vi "myRIO_BRig_RT_TCP__buildStr_initBlock.vi"(7 "input_countTrial":u16, 9 "input_spout":enum16{"Left", "Right"}(ring), 10 "input_iTrial":u16, 11 "input_iBlock":u16) -> (3 "output_str_initBlock":string)   [LabVIEW 2014]
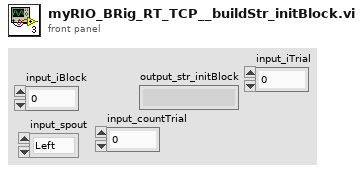
[diagram p1: front panel]
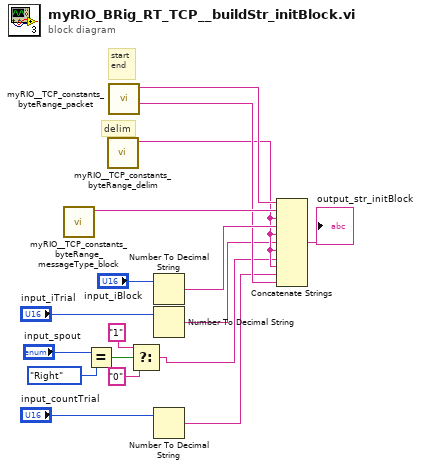
[diagram p0: block diagram]
diagram:
  # "start\nend"
  # "delim"
  n1 = call "myRIO__TCP_constants_byteRange_messageType_block.vi"() -> ("output_Block_char"=w13:string)  [unwired: 10 in, 1 out]
  n2 = Equal?(x="input_spout", y=enum16{"Left", "Right"}."Right") -> (x = y?=w4:bool)
  n3 = call "myRIO__TCP_constants_byteRange_delim.vi"() -> ("output_delim_char"=w10:string)  [unwired: 10 in, 1 out]
  n4 = call "myRIO__TCP_constants_byteRange_packet.vi"() -> ("output_end_char"=w12:string, "output_start_char"=w15:string)  [unwired: 8 in, 2 out]
  n5 = Select(t="1", s=w4, f="0") -> (s? t:f=w3:string)
  n6 = Number To Decimal String(number="input_iBlock") -> (decimal integer string=w17:string)  [unwired: 1 in]
  n7 = Number To Decimal String(number="input_iTrial") -> (decimal integer string=w7:string)  [unwired: 1 in]
  n8 = Number To Decimal String(number="input_countTrial") -> (decimal integer string=w11:string)  [unwired: 1 in]
  n9 = Concatenate Strings(w15, w13, w10, w17, w10, w7, w10, w3, w10, w11, w12) -> (→"output_str_initBlock":string)
